vi "Timestamp to string.vi"(11 "time stamp":timestamp) -> (2 "Date String":string, 3 "date/time string":string, 5 "Time String":string)   [LabVIEW 2017]
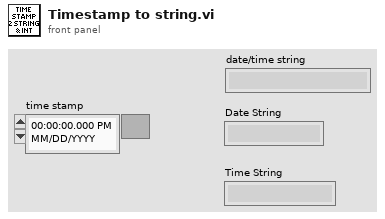
[diagram p1: front panel]
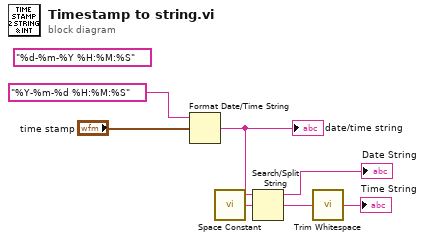
[diagram p0: block diagram]
diagram:
  (unwired) "%d-%m-%Y %H:%M:%S" ("time format string (%c)")
  n1 = Format Date/Time String(time format string (%c)="%Y-%m-%d %H:%M:%S", seconds (now)="time stamp") -> (date/time string=w2:string)  [unwired: 1 in]
  "date/time string" <- w2
  n2 = call <vilib>:"Space Constant.vi"() -> ("String"=w3:string)
  n3 = Search/Split String(string=w2, search string/char (-)=w3) -> (substring before match=→"Date String":string, match + rest of string=w5:string)  [unwired: 1 in, 1 out]
  n4 = call <vilib>:"Trim Whitespace.vi"("string"=w5) -> ("trimmed string"=→"Time String":string)  [unwired: 1 in]
